vi "Set Default.vi"(11 "Text in":refnum<class "Text.lvclass">) -> (3 "Text out":refnum<class "Text.lvclass">)   [LabVIEW 2020, in "Conditum.lvlib" / "Columns.lvlib" / "Text.lvclass"]
uses:
  Text.lvclass
  Type/Type.lvclass
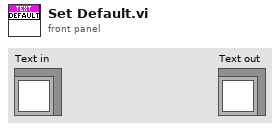
[diagram p1: front panel]
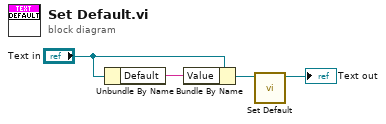
[diagram p0: block diagram]
diagram:
  n1 = Unbundle By Name("Text in") -> ("Default"=w4:string)
  n2 = Bundle By Name(cluster="Text in", "Value"=w4) -> (w3:refnum<class "Text.lvclass">)
  n3 = call-parent "Set Default.vi"("Type in"=w3) -> ("Type out"=→"Text out":refnum<class "Text.lvclass">)  [unwired: 10 in]
